vi "Read TDMS.vi"(8 "error in (no error)":errorcluster, 10 "path":path, 11 "LVtoITX in":refnum<class "LVtoITX.lvclass">) -> (0 "error out":errorcluster, 1 "Wavenames":string[](array[string]), 2 "1D Cluster Array":cluster{"array type (2D Dbl)":dbl[]}[](array[cluster]), 3 "LVtoITX out":refnum<class "LVtoITX.lvclass">, 4 "Comments":string, 6 "Igor Commands":string)   [LabVIEW 2016, in "LVtoITX.lvclass"]
uses:
  LVtoITX.lvclass
  LVtoITX.lvclass/LVtoITX.ctl
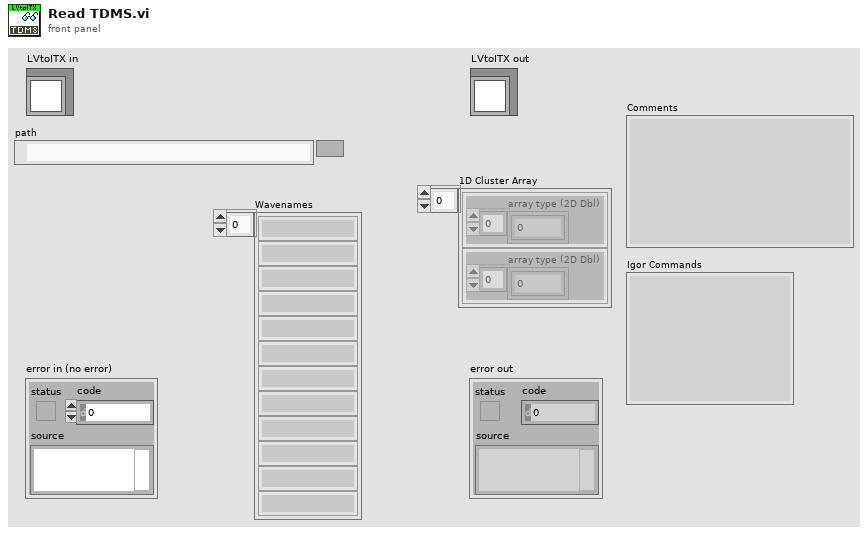
[diagram p1: front panel]
types:
  T1 = enum16{"open", "open or create", "create or replace", "create", "open (read-only)"}
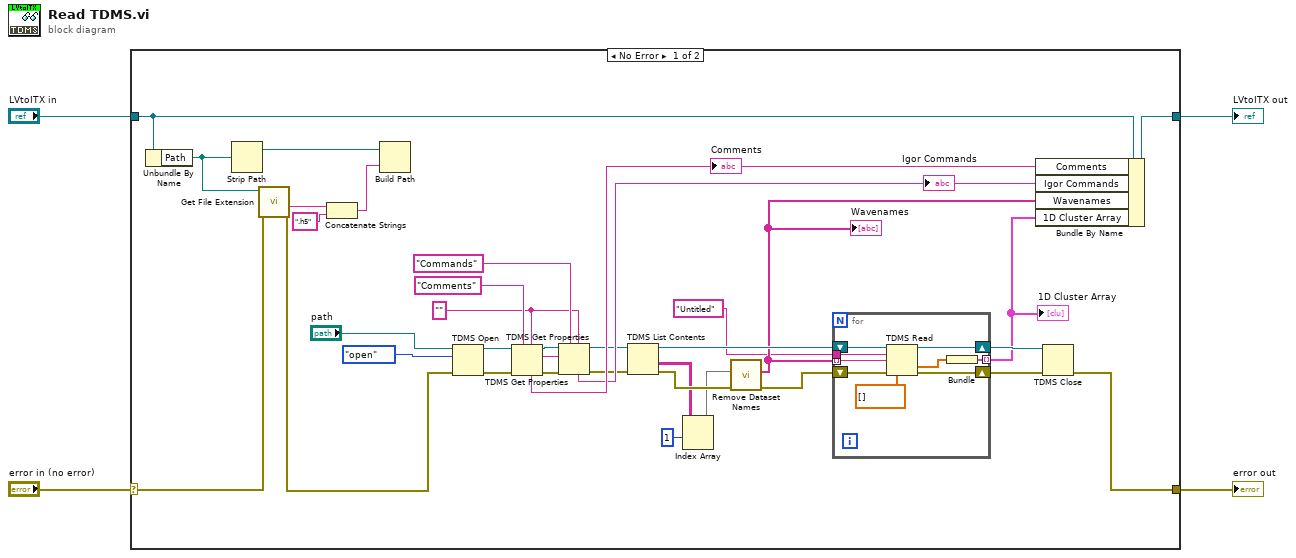
[diagram p0: block diagram]
diagram:
  n1 = case shown="No Error" "error in (no error)" {
    selector: "error in (no error)" -> [w32 w49]
    tunnel: [w18 w49] -> w1
    tunnel: [w33 w50] -> w2
    tunnel: "LVtoITX in" -> [w34 w50]
    frame No Error {
      w25 = "" ("attrib name")
      n2 = Unbundle By Name(w34) -> ("Path"=w35:path)
      n3 = Strip Path(path=w35) -> (stripped path=w37:path)  [unwired: 1 out]
      n4 = call <vilib>:"Get File Extension.vi"("error in (no error)"=w32, "file"=w35) -> ("error out"=w30:errorcluster, "filename without extension"=w39:string)  [unwired: 5 in, 3 out]
      n5 = Concatenate Strings(w39, ".h5" ("string")) -> (w36:string)
      n6 = Build Path(base path=w37, name or relative path=w36) -> ()  [unwired: 1 out]
      n7 = TDMS Open(8:w30, 10:T1."open" ("operation (0:open)"), 11:"path") -> (0:w28:errorcluster, 3:w29:refnum<k34>)  [unwired: 4 in]
      n8 = TDMS Get Properties(5:w25, 7:"Comments" ("attrib name"), 8:w28, 11:w29) -> (0:w20:errorcluster, 2:w9:string, 3:w21:refnum<k34>, 4:w24:string)  [unwired: 2 in, 2 out]
      "Comments" <- w24
      n9 = TDMS Get Properties(5:w25, 7:"Commands" ("attrib name"), 8:w20, 10:w9, 11:w21) -> (0:w19:errorcluster, 3:w22:refnum<k34>, 4:w23:string)  [unwired: 1 in, 3 out]
      "Igor Commands" <- w23
      n10 = TDMS List Contents(4:w19, 7:w22) -> (0:w11:errorcluster, 1:w6:string[][], 3:w14:refnum<k34>)  [unwired: 1 in, 1 out]
      n11 = Index Array(array=w6, index (row)=1) -> (element=w7:string[])  [unwired: 1 in]
      n12 = call "Remove Dataset Names.vi"("error in (no error)"=w11, "Dataset Names"=w7) -> ("error out"=w17:errorcluster, "Name less Commands and Comments"=w10:string[])  [unwired: 8 in]
      "Wavenames" <- w10
      n13 = for {
        tunnel: [w42] -> w12 mode=indexing
        shift-right: [w45] -> w13
        shift-left: w17 -> [w48]
        shift-right: [w47] -> w16
        shift-left: w14 -> [w46]
        tunnel: w10 -> [w41] mode=indexing
        tunnel: "Untitled" ("group name") -> [w40]
        n14 = TDMS Read(0:w46, 5:w40, 7:w41, 11:w48, 12:dbl[] [] ("array type (2D Dbl)")) -> (4:w47:refnum<k34>, 10:w43:dbl[], 15:w45:errorcluster)  [unwired: 3 in, 3 out]
        n15 = Bundle("array type (2D Dbl)"=w43) -> (w42:cluster{"array type (2D Dbl)":dbl[]})  [unwired: 1 in]
      }
      "1D Cluster Array" <- w12
      n16 = Bundle By Name(cluster=w34, "Comments"=w24, "Igor Commands"=w23, "Wavenames"=w10, "1D Cluster Array"=w12) -> (w33:refnum<class "LVtoITX.lvclass">)
      n17 = TDMS Close(8:w13, 11:w16) -> (0:w18:errorcluster)  [unwired: 1 out]
    }
    frame Error {
    }
  }
  "error out" <- w1
  "LVtoITX out" <- w2
